vi "optagefrekvenssignal0.7.vi"() -> ()   [LabVIEW 2014]
uses:
  <vilib>/measure/maspectr.llb/FFT Power Spectrum and PSD for 1 Chan.vi
  <vilib>/Utility/file.llb/Write To Spreadsheet File (DBL).vi
  <vilib>/measure/NI_MAPro.lvlib
panel:
  out "FFT af Resonansfrekvenssignal":dbl[](graph)
  out "Resonansfrekvenssignal":waveform(dbl)(graph)
  in  "Resonansfrekvens af tom resonator(f0)":dbl
  in  "Volumen af tom resonator(V)":dbl
  in  "Tid(sek)":dbl
  out "Resonansfrekvens":dbl[](array[numeric])
  out "Volumen(ml)":dbl[](array[numeric])
  # "Angivelse af nødvendige værdier til måling af brystvolumen"
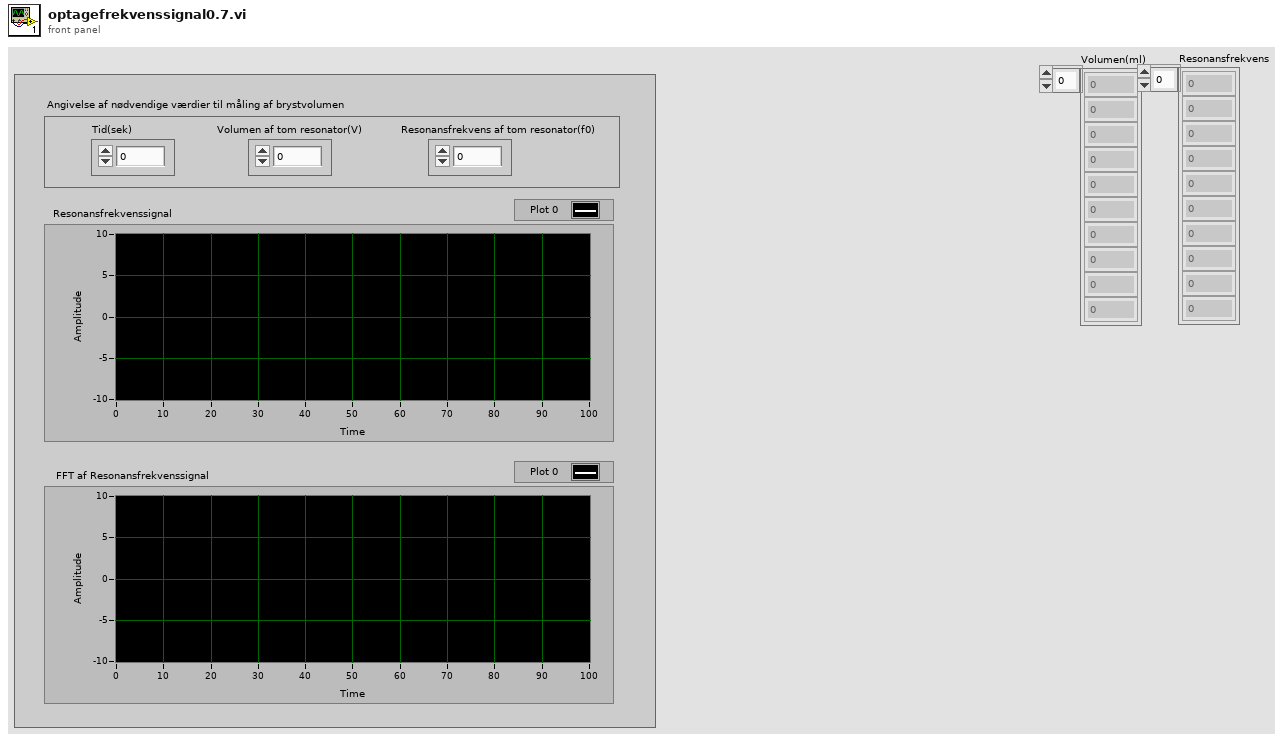
[diagram p1: front panel]
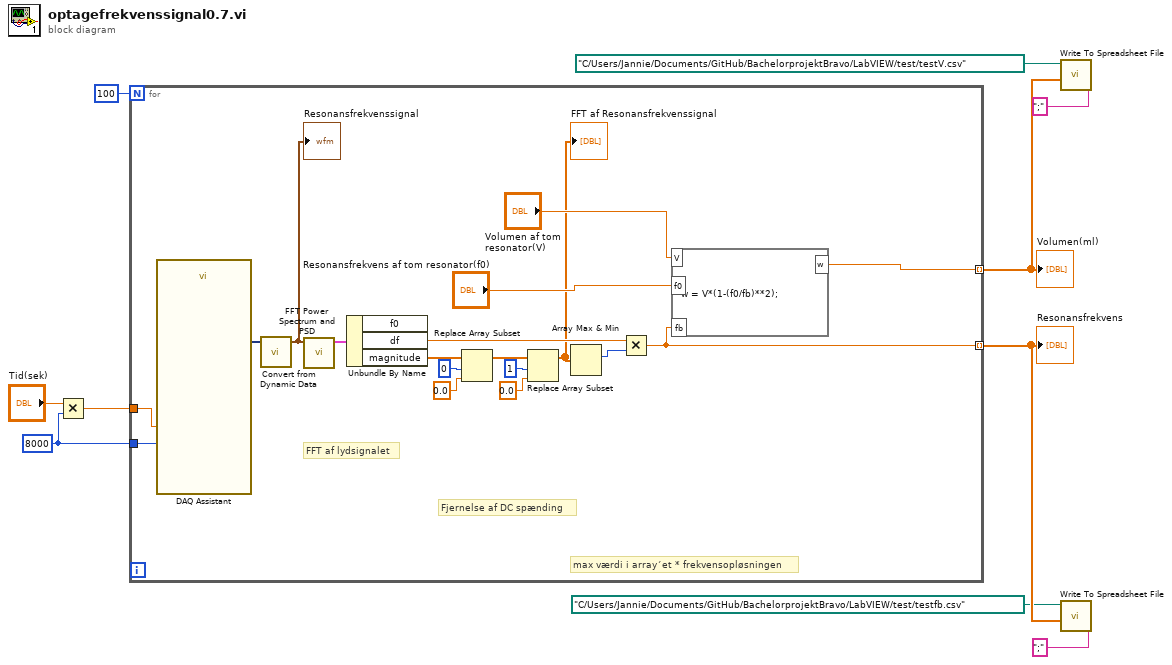
[diagram p0: block diagram]
diagram:
  w6 = 8000
  n1 = Multiply(x="Tid(sek)", y=w6) -> (x*y=w5:dbl)
  n2 = for {
    N: 100 -> [_]
    tunnel: [w19] -> w7 mode=indexing
    tunnel: [w18] -> w3 mode=indexing
    tunnel: w6 -> [w17]
    tunnel: w5 -> [w16]
    # "max værdi i array´et * frekvensopløsningen"
    # "Fjernelse af DC spænding"
    # "FFT af lydsignalet"
    n3 = call "DAQ Assistant"("rate"=w17, "number of samples"=w16) -> ("data"=w15:dynamicdata)  [unwired: 15 in, 2 out]
    n4 = call "Convert from Dynamic Data"("Dynamic Data Type"=w15) -> ("Waveform"=w11:waveform(dbl))  [unwired: 3 in]
    "Resonansfrekvenssignal" <- w11
    n5 = call-poly <vilib>:"FFT Power Spectrum and PSD.vi"("time signal"=w11) -> ("Power Spectrum / PSD"=w21:cluster{"f0":dbl, "df":dbl, "magnitude":dbl[]})  [unwired: 7 in, 3 out]
    n6 = Unbundle By Name(w21) -> ("df"=w22:dbl, "magnitude"=w20:dbl[])  [unwired: 1 out]
    n7 = Replace Array Subset(array=w20, new element=0.0 ("new element/subarray"), index=0) -> (w26:dbl[])
    n8 = Replace Array Subset(array=w26, new element=0.0 ("new element/subarray"), index=1) -> (w12:dbl[])
    "FFT af Resonansfrekvenssignal" <- w12
    n9 = Array Max & Min(array=w12) -> (max index (indices)=w23:i32)  [unwired: 3 out]
    n10 = Multiply(x=w22, y=w23) -> (x*y=w18:dbl)
    n11 = formula code="w = V*(1-(f0/fb)**2);"("V"="Volumen af tom resonator(V)", "f0"="Resonansfrekvens af tom resonator(f0)", "fb"=w18) -> ("w"=w19:dbl)
  }
  "Volumen(ml)" <- w7
  "Resonansfrekvens" <- w3
  n12 = call-poly <vilib>:"Write To Spreadsheet File.vi"("delimiter (\\t)"=";" ("delimiter (\\t)"), "1D data"=w7, "file path (dialog if empty)"=path "C:/Users/Jannie/Documents/GitHub/BachelorprojektBravo/LabVIEW/test/testV.csv") -> ()  [unwired: 5 in, 1 out]
  n13 = call-poly <vilib>:"Write To Spreadsheet File.vi"("delimiter (\\t)"=";" ("delimiter (\\t)"), "1D data"=w3, "file path (dialog if empty)"=path "C:/Users/Jannie/Documents/GitHub/BachelorprojektBravo/LabVIEW/test/testfb.csv") -> ()  [unwired: 5 in, 1 out]
